vi "Update Aliases.vi"(8 "error in (no error)":errorcluster, 11 "Valve in":refnum<class "Valve.lvclass">) -> (0 "error out":errorcluster, 3 "Valve out":refnum<class "Valve.lvclass">)   [LabVIEW 2015, in "cRIO-Carbondioxide.lvlib" / "CO2-Actor.lvlib" / "Valve.lvclass"]
uses:
  Valve.lvclass
  Valve.lvclass/Valve.ctl
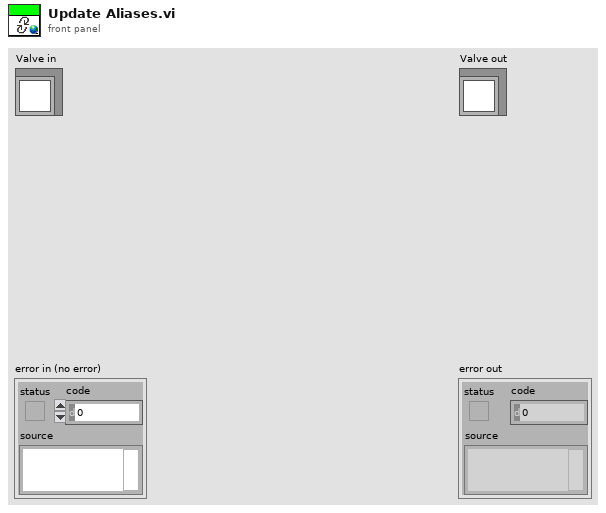
[diagram p1: front panel]
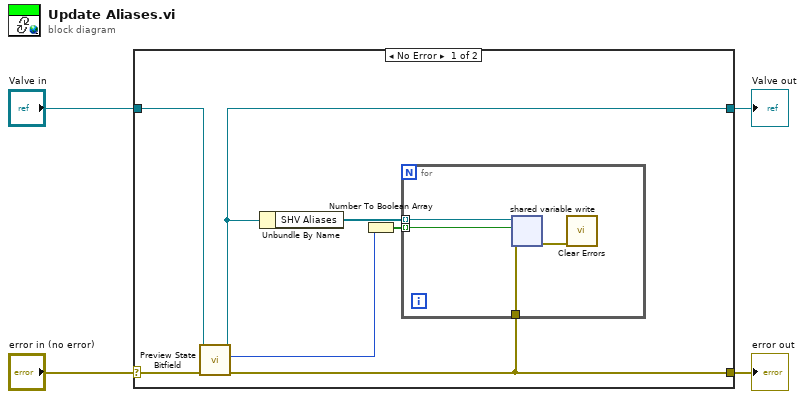
[diagram p0: block diagram]
diagram:
  n1 = case shown="No Error" "error in (no error)" {
    selector: "error in (no error)" -> [w10 w17]
    tunnel: [w5 w17] -> w3
    tunnel: [w8 w16] -> w1
    tunnel: "Valve in" -> [w9 w16]
    frame No Error {
      n2 = call "Preview State Bitfield.vi"("error in (no error)"=w10, "Valve in"=w9) -> ("error out"=w5:errorcluster, "State Bitfield"=w6:u16, "Valve out"=w8:refnum<class "Valve.lvclass">)  [unwired: 7 in]
      n3 = Unbundle By Name(w8) -> ("SHV Aliases"=w7:refnum<k21>[])
      n4 = Number To Boolean Array(number=w6) -> (Boolean array=w11:bool[])
      n5 = for {
        tunnel: w11 -> [w13] mode=indexing
        tunnel: w7 -> [w15] mode=indexing
        tunnel: w5 -> [w12]
        n6 = shared-variable-write(w15, w12, w13) -> (w14:errorcluster)  [unwired: 1 out]
        n7 = call <vilib>:"Clear Errors.vi"("error in (no error)"=w14) -> ()  [unwired: 5 in, 2 out]
      }
    }
    frame Error {
    }
  }
  "error out" <- w3
  "Valve out" <- w1
